vi "project completeRFID.vi"() -> ()   [LabVIEW 2017]
uses:
  Downloads/Compressed/ARSproj/ARSproj/ARSproj/Control 24.ctl
  <vilib>/Utility/file.llb/Read Delimited Spreadsheet (string).vi
  <vilib>/Utility/file.llb/Write Delimited Spreadsheet (string).vi
  <vilib>/Instr/_visa.llb/VISA Configure Serial Port (Instr).vi
panel:
  in  "Combo Box":string(combo)
  in  "new pass":string caption="please enter new password"
  in  "pass":string="1234"
  in  "password":bool
  in  "setting":bool
  out "number of users":i32
  in  "Cluster":T1
  out "read buffer":string
  in  "password:":string caption="enter password"
  out "MESSAGE 2":string
  out "Array":dbl[][](array[numeric])
  out "all rows":string[][](array[string])
  out "array w/ subset deleted":string[][](array[string])
  out "SERIAL ID":string
  out "FULL NAME":string
  out "PASSPORT ID":string
  out "AGE":string
  out "STUDENT NO.":string
  out "GENDER":string
  out "RACE":string
  out "BLOOD TYPE":string
  out "appended array":string[](array[string])
  out "picture3":picture
  out "error out":errorcluster
  out "MESSAGE":string
  in  "file path (text format)":path
  in  "VISA resource name":refnum<visa-resource-name>
  in  "stop":bool
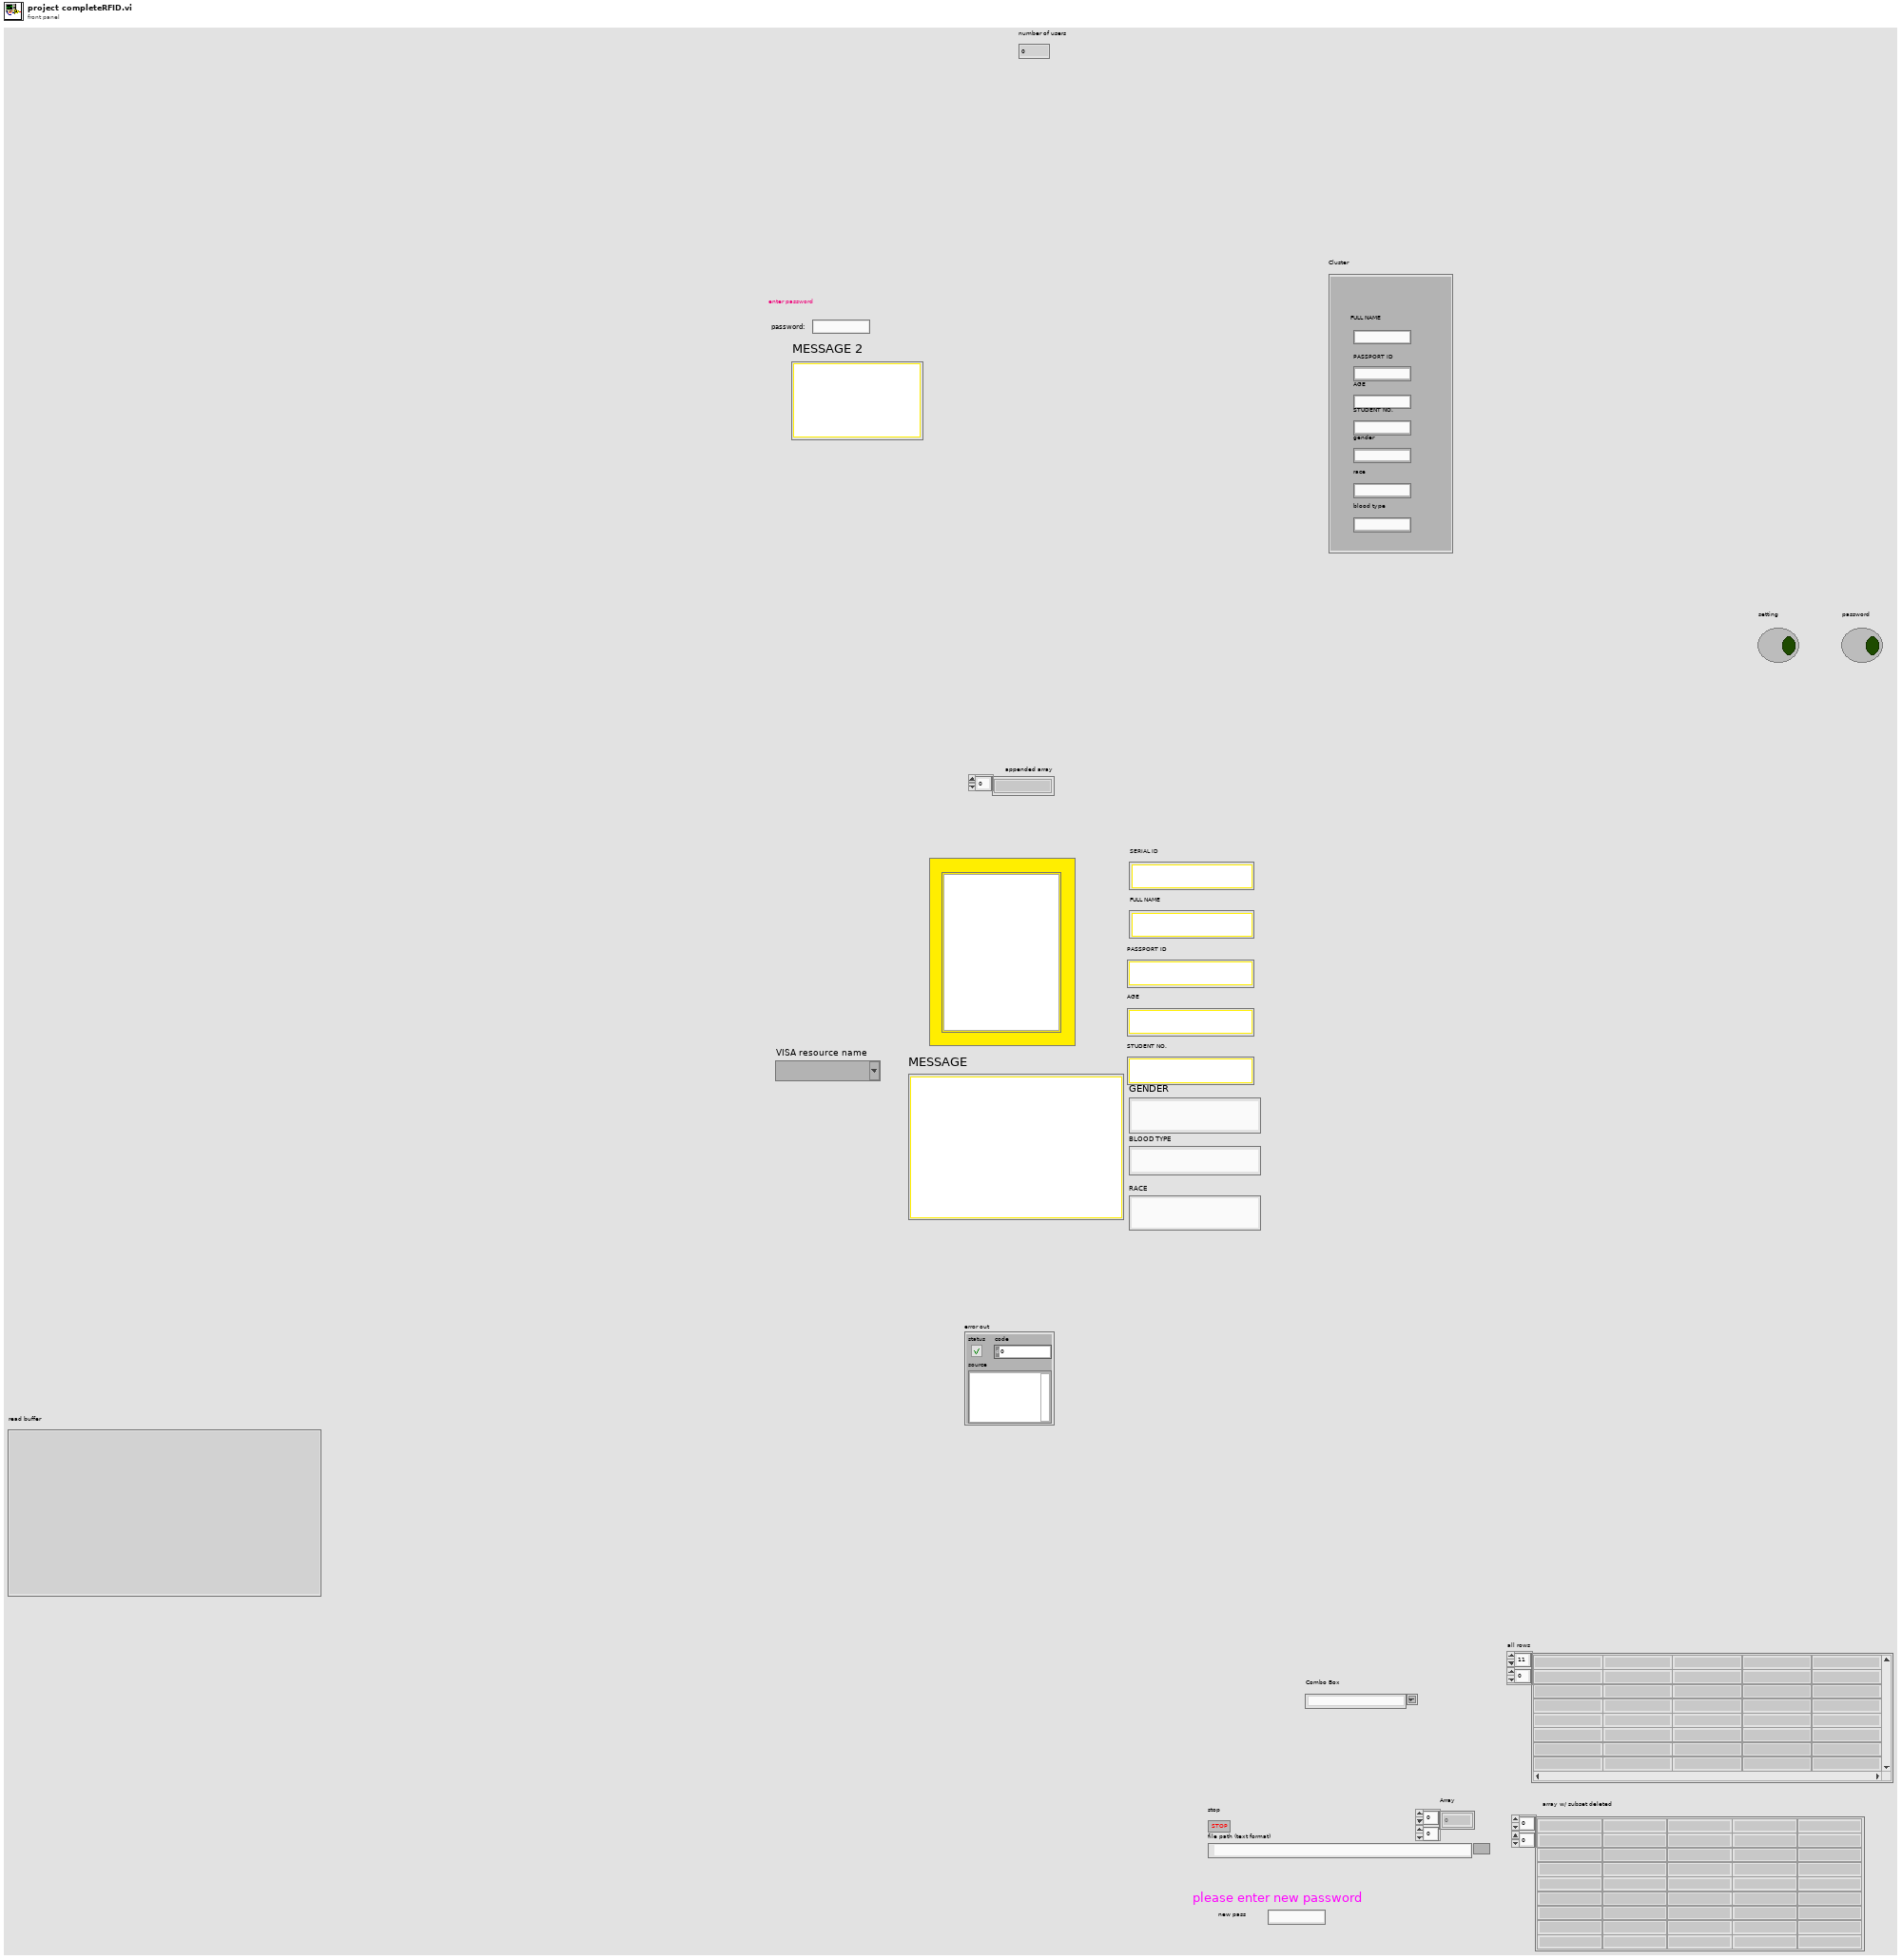
[diagram p1: front panel]
types:
  T1 = cluster{"FULL NAME":string, "PASSPORT ID":string, "AGE":string, "STUDENT NO.":string, "gender":string, "race":string, "blood type":string}
  T2 = typedef "Control 24.ctl" = enum32{"default", "checkin", "register", "stop"}
  T3 = cluster{"all rows[0]":string, "all rows[1]":string, "all rows[2]":string, "all rows[3]":string, "all rows[4]":string, "all rows[5]":string, "all rows[6]":string, "all rows[7]":string, "all rows[8]":string}
  T4 = typedef "imagedata.ctl" = cluster{"image type":i32, "image depth":i32, "image":u8[], "mask":u8[], "colors":u32[], "Rectangle":cluster{"left":i16, "top":i16, "right":i16, "bottom":i16}}
  T5 = cluster{string, string, string, string, string, string, string}
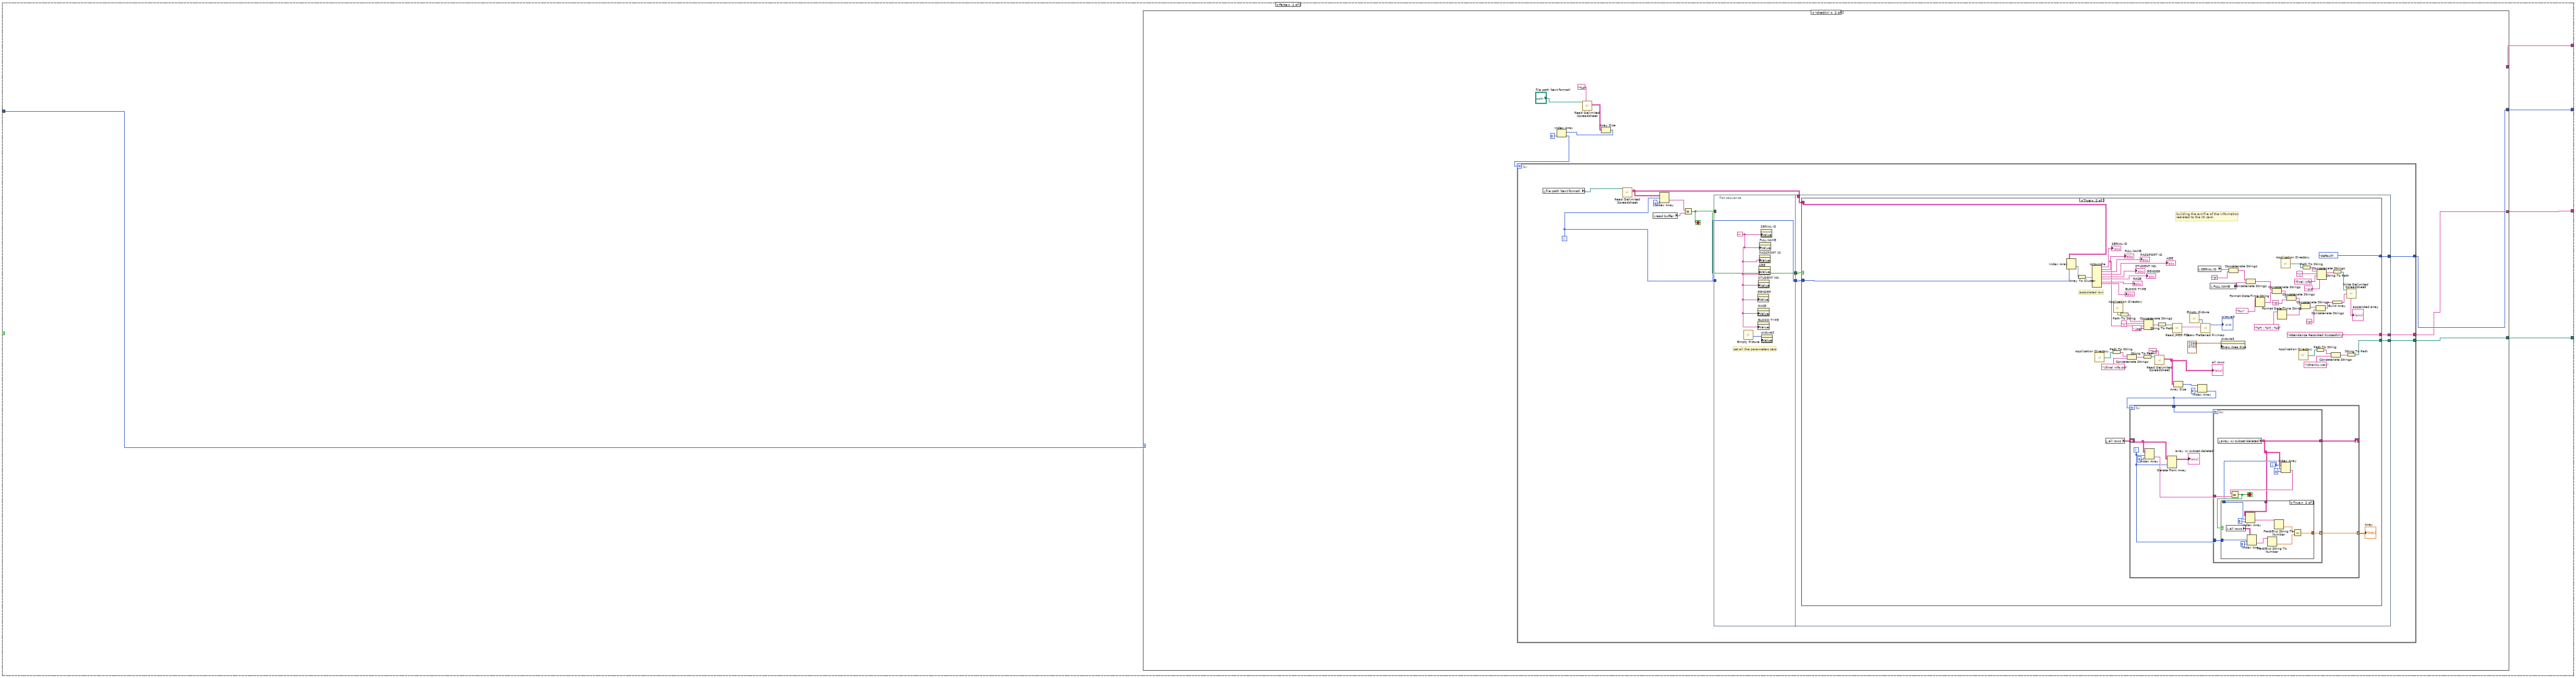
[diagram p2: hidden frame]
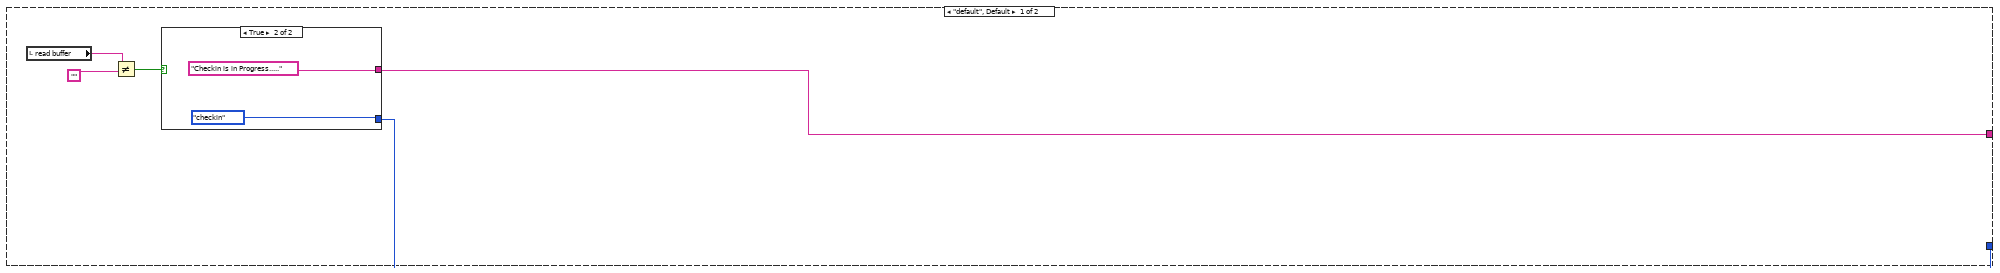
[diagram p3: hidden frame]
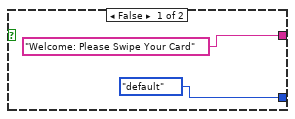
[diagram p4: hidden frame]
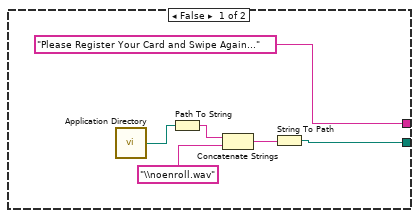
[diagram p5: hidden frame]
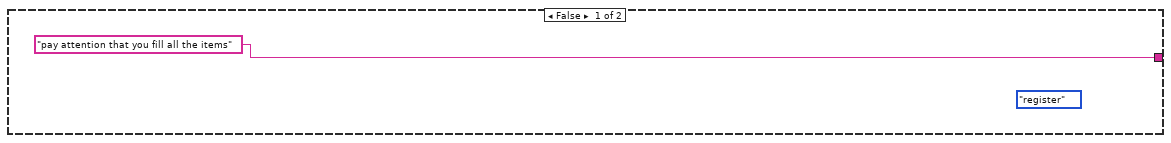
[diagram p8: hidden frame]
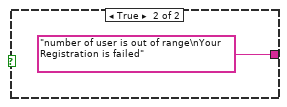
[diagram p9: hidden frame]
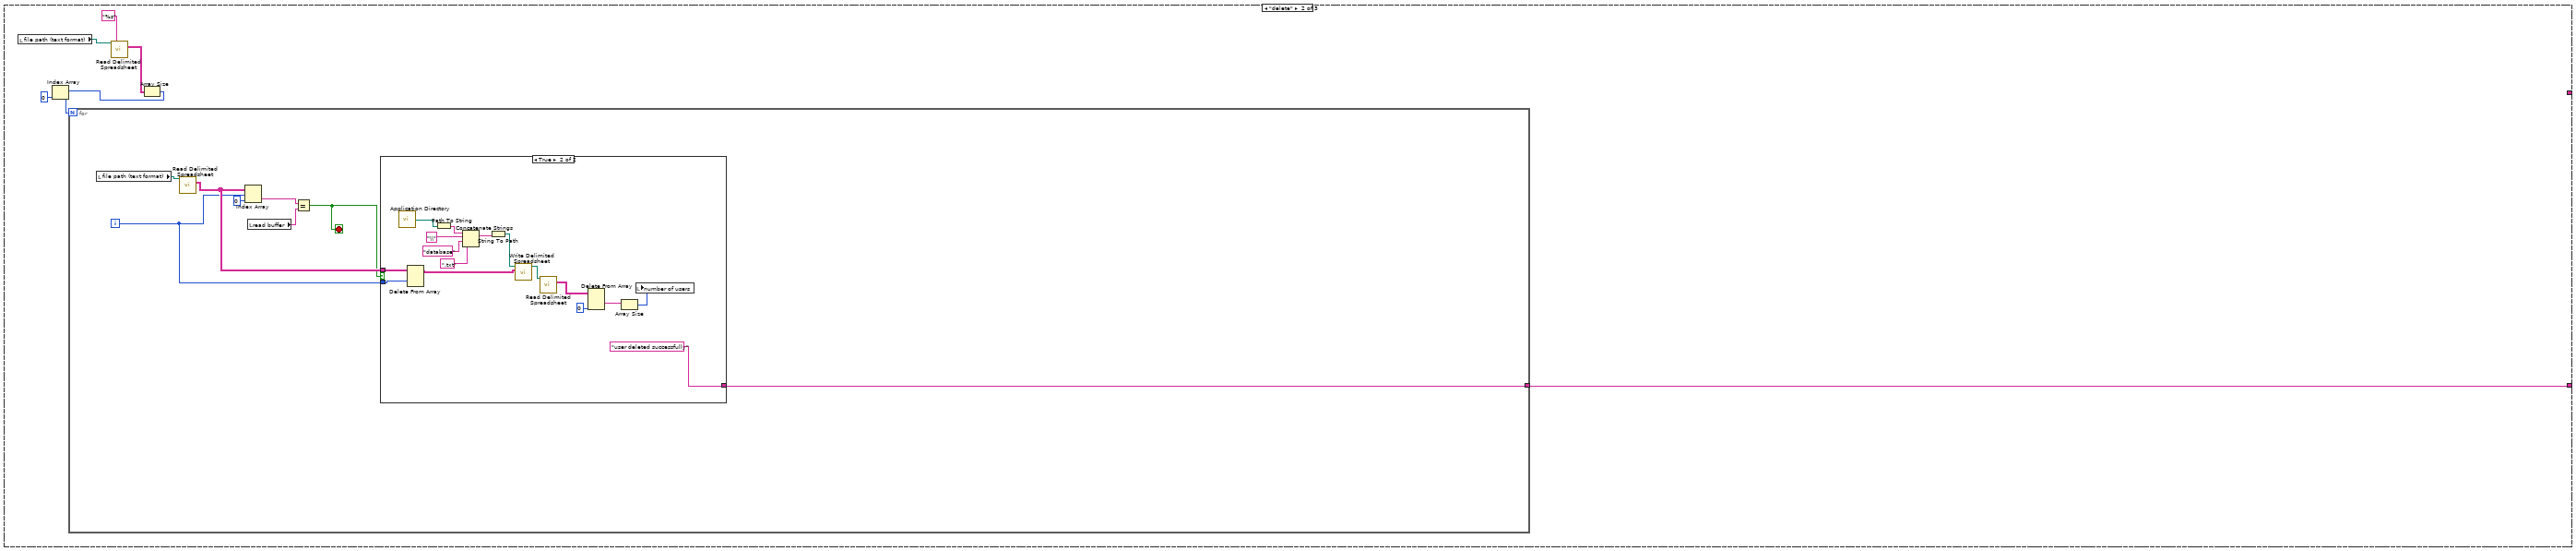
[diagram p10: hidden frame]
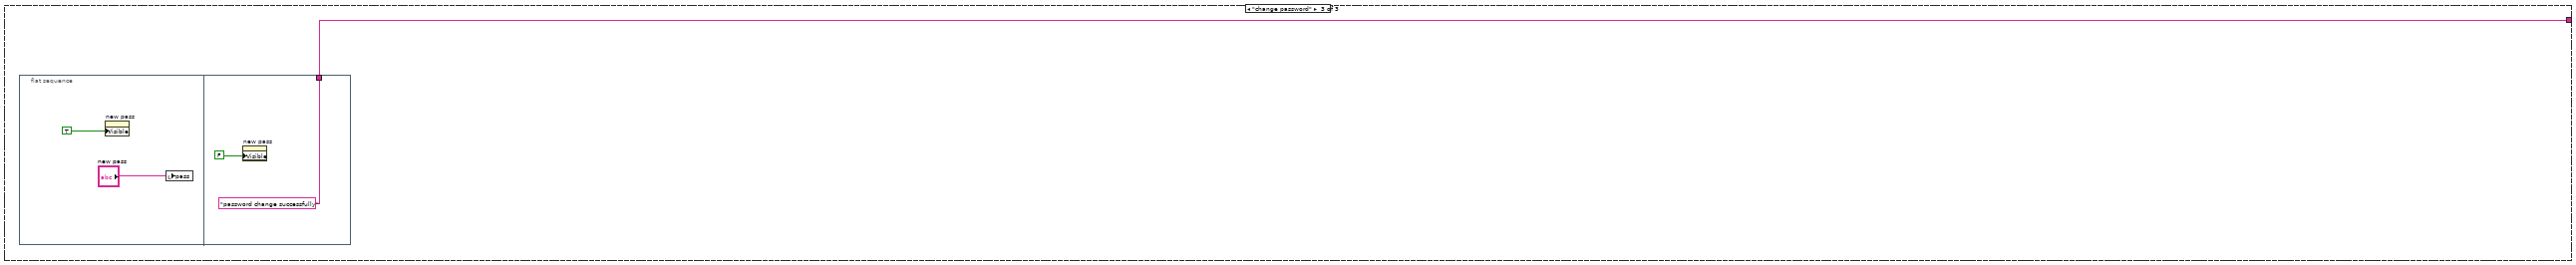
[diagram p12: hidden frame]
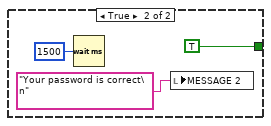
[diagram p16: hidden frame]
diagram:
  n1 = call-poly "VISA Configure Serial Port"("VISA resource name"="VISA resource name") -> ("VISA resource name out"=w1:refnum<visa-resource-name>, "error out"=w2:errorcluster)  [unwired: 13 in]
  n2 = while {
    shift-right: [w24] -> _
    shift-left: Control_24."default" ("Enum") -> [w25]
    shift-right: [w22] -> w3
    shift-left: w1 -> [w8]
    shift-right: [w23] -> w4
    shift-left: w2 -> [w13]
    stop <- "stop" stop-if-true
    n3 = property class="Instr"(reference=w8, error in=w13, "General Settings:Timeout Value"=u32 2000) -> (reference out=w18:refnum<visa-resource-name>, error out=w17:errorcluster)
    n4 = VISA Write(VISA resource name=w18, write buffer="%IDN?", error in (no error)=w17) -> (VISA resource name out=w15:refnum<visa-resource-name>, error out=w21:errorcluster)  [unwired: 1 out]
    n5 = VISA Read(VISA resource name=w15, byte count=u32 11, error in (no error)=w21) -> (VISA resource name out=w22:refnum<visa-resource-name>, read buffer=→"read buffer":string, error out=w23:errorcluster)  [unwired: 1 out]
    n6 = case shown="True" "setting" {
      tunnel: w25 -> [w31 _]
      tunnel: [w30 _] -> w24
      tunnel: [w29 w169] -> w14
      tunnel: [w28 w171] -> w12
      tunnel: [w27 _] -> w11
      frame False {
        n7 = case shown="\"checkin\"" w31 {
          tunnel: [w32 w49] -> w30
          tunnel: [w33 _] -> w29
          tunnel: [_ w48] -> w28
          tunnel: [_ w47] -> w27
          frame "default", Default {
            n8 = local read "read buffer"() -> (w35:string)
            n9 = Not Equal?(x=w35, y="") -> (x != y?=w34:bool)
            n10 = case shown="True" w34 {
              tunnel: ["Welcome: Please Swipe Your Card" "Checkin is in Progress....." ("write buffer")] -> w33
              tunnel: [Control_24."default" ("Enum") Control_24."checkin" ("Enum")] -> w32
              frame False {
              }
              frame True {
              }
            }
          }
          frame "checkin" {
            n11 = call-poly <vilib>:"Read Delimited Spreadsheet.vi"("file path (dialog if empty)"="file path (text format)", "format (%s)"="%s" ("format (%.3f)")) -> ("all rows"=w44:string[][])  [unwired: 8 in, 5 out]
            n12 = Array Size(array=w44) -> (size(s)=w46:i32[])
            n13 = Index Array(array=w46, index=0) -> (element=w41:i32)
            n14 = for {
              N: w41 -> [_]
              tunnel: [w53] -> w48
              tunnel: [w52] -> w47
              tunnel: [w51] -> w49
              i -> [w54]
              stop <- w57 stop-if-true
              n15 = local read "file path (text format)"() -> (w50:path)
              n16 = call-poly <vilib>:"Read Delimited Spreadsheet.vi"("file path (dialog if empty)"=w50) -> ("all rows"=w56:string[][])  [unwired: 9 in, 5 out]
              n17 = local read "read buffer"() -> (w55:string)
              n18 = Index Array(array=w56, index (row)=w54, index (col)=0 ("disabled index (col)")) -> (element=w60:string)
              n19 = Equal?(x=w60, y=w55) -> (x = y?=w57:bool)
              n20 = flat-sequence {
                tunnel: w54 -> [w65]
                tunnel: [w62] -> w59
                tunnel: [w65] -> w58
                tunnel: w57 -> [w62]
                tunnel: w56 -> [w71]
                tunnel: w59 -> [w70]
                tunnel: w58 -> [w69]
                tunnel: [w68] -> w53
                tunnel: [w67] -> w52
                tunnel: [w66] -> w51
                frame #0 {
                  w63 = ""
                  # "set all the parameters zero"
                  n21 = call "Empty Picture"() -> ("empty picture"=w64:picture)
                  n22 = property on="GENDER" class="Str"("Value"=w63) -> ()  [unwired: 2 in, 2 out]
                  n23 = property on="RACE" class="Str"("Value"=w63) -> ()  [unwired: 2 in, 2 out]
                  n24 = property on="BLOOD TYPE" class="Str"("Value"=w63) -> ()  [unwired: 2 in, 2 out]
                  n25 = property on="STUDENT NO." class="Str"("Value"=w63) -> ()  [unwired: 2 in, 2 out]
                  n26 = property on="AGE" class="Str"("Value"=w63) -> ()  [unwired: 2 in, 2 out]
                  n27 = property on="PASSPORT ID" class="Str"("Value"=w63) -> ()  [unwired: 2 in, 2 out]
                  n28 = property on="FULL NAME" class="Str"("Value"=w63) -> ()  [unwired: 2 in, 2 out]
                  n29 = property on="SERIAL ID" class="Str"("Value"=w63) -> ()  [unwired: 2 in, 2 out]
                  n30 = property on="picture3" class="Pict"("Value"=w64) -> ()  [unwired: 2 in, 2 out]
                }
                frame #1 {
                  n31 = case shown="True" w70 {
                    tunnel: w71 -> [_ w141]
                    tunnel: w69 -> [_ w140]
                    tunnel: ["Please Register Your Card and Swipe Again..." ("format (%.3f)") "Attendance Recorded Succesfully" ("format (%.3f)")] -> w68
                    tunnel: [w72 w137] -> w67
                    tunnel: [_ Control_24."default" ("Enum")] -> w66
                    frame False {
                      n32 = call <vilib>:"Application Directory.vi"() -> ("Application Directory"=w74:path)
                      n33 = Path To String(path=w74) -> (string=w77:string)
                      n34 = Concatenate Strings(w77, "\\noenroll.wav") -> (w75:string)
                      n35 = String To Path(string=w75) -> (path=w72:path)
                    }
                    frame True {
                      # "building the ext file of the information\nrealated to the ID card."
                      # "associated row"
                      n36 = Index Array(array=w141, index (row)=w140) -> (element=w136:string[])  [unwired: 1 in]
                      n37 = Array To Cluster(array=w136) -> (cluster=w131:T3)
                      n38 = Unbundle(w131) -> ("all rows[0]"=→"SERIAL ID":string, "all rows[1]"=w103:string, "all rows[2]"=→"PASSPORT ID":string, "all rows[3]"=→"AGE":string, "all rows[4]"=→"STUDENT NO.":string, "all rows[5]"=→"GENDER":string, "all rows[6]"=→"RACE":string, "all rows[7]"=→"BLOOD TYPE":string)  [unwired: 1 out]
                      "FULL NAME" <- w103
                      n39 = call <vilib>:"Application Directory.vi"() -> ("Application Directory"=w84:path)
                      n40 = local read "all rows"() -> (w97:string[][])
                      n41 = Path To String(path=w84) -> (string=w87:string)
                      n42 = call <vilib>:"Application Directory.vi"() -> ("Application Directory"=w107:path)
                      n43 = Path To String(path=w107) -> (string=w108:string)
                      n44 = Concatenate Strings(w87, "\\final info.txt") -> (w85:string)
                      n45 = String To Path(string=w85) -> (path=w83:path)
                      n46 = Concatenate Strings(w108, "\\" ("string"), w103, ".jpg" ("string")) -> (w105:string)
                      n47 = call-poly <vilib>:"Read Delimited Spreadsheet.vi"("file path (dialog if empty)"=w83, "format (%s)"="%s" ("format (%.3f)")) -> ("all rows"=w98:string[][])  [unwired: 8 in, 5 out]
                      "all rows" <- w98
                      n48 = String To Path(string=w105) -> (path=w109:path)
                      n49 = call <vilib>:"Read JPEG File.vi"("path to JPEG file"=w109) -> ("image data"=w112:T4)  [unwired: 8 in, 2 out]
                      n50 = Array Size(array=w98) -> (size(s)=w78:i32[])
                      n51 = call "Empty Picture"() -> ("empty picture"=w110:picture)
                      n52 = Index Array(array=w78, index=0) -> (element=w99:i32)
                      n53 = for {
                        N: w99 -> [_]
                        tunnel: w99 -> [w148]
                        shift-right: [w143] -> _
                        shift-left: w97 -> [w144]
                        tunnel: [w142] -> w80 mode=indexing
                        i -> [w145]
                        n54 = Index Array(array=w144, index (row)=w145, index (col)=0 ("disabled index (col)")) -> (element=w146:string)
                        n55 = Delete From Array(array=w144, index (row)=w145) -> (array with subset deleted=→"array w/ subset deleted":string[][])  [unwired: 2 in, 1 out]
                        n56 = for {
                          N: w148 -> [_]
                          tunnel: w146 -> [w155]
                          tunnel: w145 -> [w152]
                          tunnel: [w151] -> w142 mode=indexing
                          tunnel: [w150] -> w143
                          i -> [w153]
                          stop <- w154 stop-if-true
                          n57 = local read "array w/ subset deleted"() -> (w150:string[][])
                          n58 = Index Array(array=w150, index (row)=w153, index (col)=0 ("disabled index (col)")) -> (element=w156:string)
                          n59 = Equal?(x=w156, y=w155) -> (x = y?=w154:bool)
                          n60 = case shown="True" w154 {
                            tunnel: w153 -> [_ w167]
                            tunnel: w150 -> [_ w164]
                            tunnel: w152 -> [_ w165]
                            tunnel: [_ w160] -> w151
                            frame False {
                            }
                            frame True {
                              n61 = local read "all rows"() -> (w159:string[][])
                              n62 = Index Array(array=w164, index (row)=w167, index (col)=9) -> (element=w158:string)
                              n63 = Index Array(array=w159, index (row)=w165, index (col)=9) -> (element=w163:string)
                              n64 = Fract/Exp String To Number(string=w163) -> (number=w161:dbl)  [unwired: 3 in, 1 out]
                              n65 = Fract/Exp String To Number(string=w158) -> (number=w162:dbl)  [unwired: 3 in, 1 out]
                              n66 = Subtract(x=w162, y=w161) -> (x-y=w160:dbl)
                            }
                          }
                        }
                      }
                      "Array" <- w80
                      n67 = local read "SERIAL ID"() -> (w126:string)
                      n68 = call <vilib>:"Draw Flattened Pixmap.vi"("image data"=w112, "picture"=w110) -> ("new picture"=→"picture3":picture)  [unwired: 7 in]
                      n69 = local read "FULL NAME"() -> (w123:string)
                      n70 = property on="picture3" class="Pict"("Draw Area Size"=cluster{"Width":u32, "Height":u32} {"Width"=200, "Height"=270}) -> ()  [unwired: 2 in, 2 out]
                      n71 = Concatenate Strings(w126, "\t") -> (w124:string)
                      n72 = Concatenate Strings(w124, w123) -> (w79:string)
                      n73 = Format Date/Time String(time format string (%c)="%x") -> (date/time string=w117:string)  [unwired: 2 in]
                      n74 = Concatenate Strings(w79, w117) -> (w122:string)
                      n75 = Format Date/Time String(time format string (%c)="%H : %M : %S") -> (date/time string=w118:string)  [unwired: 2 in]
                      n76 = call <vilib>:"Application Directory.vi"() -> ("Application Directory"=w89:path)
                      n77 = Concatenate Strings(w122, "\t") -> (w121:string)
                      n78 = call <vilib>:"Application Directory.vi"() -> ("Application Directory"=w93:path)
                      n79 = Concatenate Strings(w121, w118) -> (w120:string)
                      n80 = Path To String(path=w89) -> (string=w92:string)
                      n81 = Path To String(path=w93) -> (string=w96:string)
                      n82 = Concatenate Strings(w120, "\t") -> (w114:string)
                      n83 = Concatenate Strings(w92, "\\", "final info" ("string"), ".txt" ("string")) -> (w90:string)
                      n84 = Concatenate Strings(w96, "\\thanku.wav") -> (w94:string)
                      n85 = String To Path(string=w90) -> (path=w88:path)
                      n86 = Build Array(w114) -> (w127:string[])
                      "appended array" <- w127
                      n87 = String To Path(string=w94) -> (path=w137:path)
                      n88 = call-poly <vilib>:"Write Delimited Spreadsheet.vi"("file path (dialog if empty)"=w88, "1D data"=w127) -> ()  [unwired: 12 in, 2 out]
                    }
                  }
                }
              }
            }
          }
        }
      }
      frame True {
        n89 = case shown="True" "password" {
          selector: "password" -> [_ w292]
          tunnel: [_ w291] -> w172
          frame False {
          }
          frame True {
            n90 = for {
              N: 4 -> [_]
              tunnel: "pass" -> [w302]
              tunnel: w292 -> [w297]
              tunnel: [w295] -> w291
              i -> [w300]
              stop <- w295 stop-if-true
              n91 = property on="password:" class="Str"("Visible"=w297) -> ()  [unwired: 2 in, 2 out]
              n92 = flat-sequence {
                tunnel: ["password:"] -> w301
                tunnel: w301 -> [w313]
                tunnel: w302 -> [w315]
                tunnel: [w311] -> w295
                frame #0 {
                  n93 = Wait (ms)(milliseconds to wait=u32 5000) -> ()  [unwired: 1 out]
                }
                frame #1 {
                  n94 = property on="password:" class="Str"("Visible"=FALSE) -> ()  [unwired: 2 in, 2 out]
                  n95 = Wait (ms)(milliseconds to wait=u32 1000) -> ()  [unwired: 1 out]
                }
                frame #2 {
                  n96 = Equal?(x=w313, y="") -> (x = y?=w312:bool)
                  n97 = case shown="False" w312 {
                    tunnel: [w319 _] -> w311
                    tunnel: w315 -> [w318 _]
                    tunnel: w313 -> [w316 _]
                    frame False {
                      n98 = Equal?(x=w316, y=w318) -> (x = y?=w317:bool)
                      n99 = case shown="False" w317 {
                        tunnel: [_ TRUE] -> w319
                        frame False {
                          n100 = Wait (ms)(milliseconds to wait=u32 1000) -> ()  [unwired: 1 out]
                          n101 = property on="password:" class="Str"("Value"="") -> ()  [unwired: 2 in, 2 out]
                          n102 = local write "MESSAGE 2"("Your password is incorrect") -> ()
                        }
                        frame True {
                          n103 = Wait (ms)(milliseconds to wait=u32 1500) -> ()  [unwired: 1 out]
                          n104 = local write "MESSAGE 2"("Your password is correct\n") -> ()
                        }
                      }
                    }
                    frame True {
                    }
                  }
                }
              }
              n105 = Equal?(x=3, y=w300) -> (x = y?=w296:bool)
              n106 = case shown="True" w296 {
                frame False {
                }
                frame True {
                  n107 = local write "setting"(FALSE) -> ()
                  n108 = local write "MESSAGE 2"("") -> ()
                }
              }
              n109 = case shown="True" w295 {
                frame False {
                }
                frame True {
                  n110 = local write "MESSAGE 2"("") -> ()
                  n111 = local write "password"(FALSE) -> ()
                }
              }
              "MESSAGE 2" <- ""
            }
          }
        }
        n112 = case shown="True" w172 {
          tunnel: [_ w175] -> w171
          tunnel: [_ w174] -> w169
          frame False {
          }
          frame True {
            n113 = case shown="\"register\", Default" "Combo Box" {
              tunnel: [w176 w255 _] -> w175
              tunnel: [_ _ w286] -> w174
              frame "register", Default {
                w177 = ""
                n114 = Bundle(w177, w177, w177, w177, w177, w177, w177) -> (w179:T5)  [unwired: 1 in]
                n115 = property on="Cluster" class="Clust (strict)"("Visible"=TRUE) -> ()  [unwired: 2 in, 2 out]
                n116 = local write "Cluster"(w179) -> ()
                n117 = Unbundle("Cluster") -> ("FULL NAME"=w186:string, "PASSPORT ID"=w185:string, "AGE"=w184:string, "STUDENT NO."=w183:string, "gender"=w182:string, "race"=w181:string, "blood type"=w180:string)
                n118 = Not Equal?(x=w183, y="") -> (x != y?=w191:bool)
                n119 = Not Equal?(x=w185, y="") -> (x != y?=w193:bool)
                n120 = Not Equal?(x=w182, y="") -> (x != y?=w190:bool)
                n121 = Not Equal?(x=w186, y="") -> (x != y?=w194:bool)
                n122 = Not Equal?(x=w184, y="") -> (x != y?=w192:bool)
                n123 = Not Equal?(x=w181, y="") -> (x != y?=w189:bool)
                n124 = Not Equal?(x=w180, y="") -> (x != y?=w188:bool)
                n125 = Compound Arithmetic op=AND(w194, w193, w192, w191, w190, w189, w188) -> (w187:bool)  [unwired: 1 in]
                n126 = case shown="True" w187 {
                  tunnel: ["pay attention that you fill all the items" w230] -> w176
                  tunnel: w185 -> [_ w220]
                  tunnel: w184 -> [_ w219]
                  tunnel: w183 -> [_ w218]
                  tunnel: w186 -> [_ w217]
                  tunnel: w182 -> [_ w216]
                  tunnel: w181 -> [_ w215]
                  tunnel: w180 -> [_ w214]
                  frame False {
                    w203 = enum16{"change password", "delete", "register"}."register" ("Enum 2")
                  }
                  frame True {
                    w210 = "\t"
                    n127 = local read "read buffer"() -> (w206:string)
                    n128 = Concatenate Strings(w206, "\t") -> (w249:string)
                    n129 = Concatenate Strings(w249, w217) -> (w248:string)
                    n130 = Concatenate Strings(w248, "\t") -> (w246:string)
                    n131 = Concatenate Strings(w246, w220) -> (w245:string)
                    n132 = Concatenate Strings(w245, "\t") -> (w212:string)
                    n133 = Concatenate Strings(w212, w219) -> (w243:string)
                    n134 = Concatenate Strings(w243, w210) -> (w242:string)
                    n135 = Concatenate Strings(w242, w218) -> (w211:string)
                    n136 = Concatenate Strings(w211, w210) -> (w209:string)
                    n137 = Concatenate Strings(w209, w216) -> (w229:string)
                    n138 = Concatenate Strings(w229, "\t") -> (w225:string)
                    n139 = Concatenate Strings(w225, w215) -> (w227:string)
                    n140 = Concatenate Strings(w227, "\t") -> (w222:string)
                    n141 = call <vilib>:"Application Directory.vi"() -> ("Application Directory"=w238:path)
                    n142 = Concatenate Strings(w222, w214) -> (w224:string)
                    n143 = Path To String(path=w238) -> (string=w241:string)
                    n144 = Concatenate Strings(w241, "\\", "database" ("string"), ".txt" ("string")) -> (w239:string)
                    n145 = Concatenate Strings(w224, "\t") -> (w221:string)
                    n146 = Build Array(w221) -> (w251:string[])
                    n147 = String To Path(string=w239) -> (path=w237:path)
                    n148 = call-poly <vilib>:"Write Delimited Spreadsheet.vi"("file path (dialog if empty)"=w237, "format (%s)"="%s" ("format (%.3f)"), "1D data"=w251, "delimiter (\\t)"="/t" ("delimiter (\\t)")) -> ("new file path (Not A Path if cancelled)"=w234:path)  [unwired: 10 in, 1 out]
                    n149 = call-poly <vilib>:"Read Delimited Spreadsheet.vi"("file path (dialog if empty)"=w234) -> ("all rows"=w233:string[][])  [unwired: 9 in, 5 out]
                    n150 = Delete From Array(array=w233, index (col)=0 ("disabled index (col)")) -> (deleted portion=w235:string[])  [unwired: 2 in, 1 out]
                    n151 = Array Size(array=w235) -> (size(s)=w231:i32)
                    "number of users" <- w231
                    n152 = Greater?(x=w231, y=50) -> (0:w213:bool)
                    n153 = case shown="False" w213 {
                      tunnel: ["Your Registration Success" ("write buffer") "number of user is out of range\nYour Registration is failed" ("write buffer")] -> w230
                      frame False {
                      }
                      frame True {
                      }
                    }
                  }
                }
              }
              frame "delete" {
                n154 = local read "file path (text format)"() -> (w257:path)
                n155 = call-poly <vilib>:"Read Delimited Spreadsheet.vi"("file path (dialog if empty)"=w257, "format (%s)"="%s" ("format (%.3f)")) -> ("all rows"=w259:string[][])  [unwired: 8 in, 5 out]
                n156 = Array Size(array=w259) -> (size(s)=w261:i32[])
                n157 = Index Array(array=w261, index=0) -> (element=w256:i32)
                n158 = for {
                  N: w256 -> [_]
                  tunnel: [w262] -> w255
                  i -> [w263]
                  stop <- w264 stop-if-true
                  n159 = local read "file path (text format)"() -> (w269:path)
                  n160 = call-poly <vilib>:"Read Delimited Spreadsheet.vi"("file path (dialog if empty)"=w269) -> ("all rows"=w267:string[][])  [unwired: 9 in, 5 out]
                  n161 = Index Array(array=w267, index (row)=w263, index (col)=0 ("disabled index (col)")) -> (element=w266:string)
                  n162 = local read "read buffer"() -> (w265:string)
                  n163 = Equal?(x=w266, y=w265) -> (x = y?=w264:bool)
                  n164 = case shown="True" w264 {
                    tunnel: w267 -> [_ w272]
                    tunnel: w263 -> [_ w271]
                    tunnel: [_ "user deleted successfully"] -> w262
                    frame False {
                    }
                    frame True {
                      n165 = call <vilib>:"Application Directory.vi"() -> ("Application Directory"=w282:path)
                      n166 = Delete From Array(array=w272, index (row)=w271) -> (array with subset deleted=w278:string[][])  [unwired: 2 in, 1 out]
                      n167 = Path To String(path=w282) -> (string=w285:string)
                      n168 = Concatenate Strings(w285, "\\", "database" ("string"), ".txt" ("string")) -> (w283:string)
                      n169 = String To Path(string=w283) -> (path=w281:path)
                      n170 = call-poly <vilib>:"Write Delimited Spreadsheet.vi"("file path (dialog if empty)"=w281, "2D data"=w278) -> ("new file path (Not A Path if cancelled)"=w275:path)  [unwired: 12 in, 1 out]
                      n171 = call-poly <vilib>:"Read Delimited Spreadsheet.vi"("file path (dialog if empty)"=w275) -> ("all rows"=w276:string[][])  [unwired: 9 in, 5 out]
                      n172 = Delete From Array(array=w276, index (col)=0 ("disabled index (col)")) -> (deleted portion=w277:string[])  [unwired: 2 in, 1 out]
                      n173 = Array Size(array=w277) -> (size(s)=w274:i32)
                      n174 = local write "number of users"(w274) -> ()
                    }
                  }
                }
              }
              frame "change password" {
                n175 = flat-sequence {
                  tunnel: ["password change successfully"] -> w286
                  frame #0 {
                    n176 = property on="new pass" class="Str"("Visible"=TRUE) -> ()  [unwired: 2 in, 2 out]
                    n177 = local write "pass"("new pass") -> ()
                  }
                  frame #1 {
                    n178 = property on="new pass" class="Str"("Visible"=FALSE) -> ()  [unwired: 2 in, 2 out]
                  }
                }
              }
            }
          }
        }
      }
    }
    "MESSAGE" <- w14
    n179 = local write "MESSAGE"(w12) -> ()
    n180 = call <vilib>:"Play Sound File.vi"("path"=w11) -> ()  [unwired: 9 in, 2 out]
  }
  n181 = VISA Close(VISA resource name=w3, error in (no error)=w4) -> (error out=→"error out":errorcluster)
